vi "Swerve Global Variables.vi"() -> ()   [LabVIEW 2020]
doc: "Global variables in charge of the Swerve Drive subsystem."
panel:
  in  "Target Extension":dbl
  in  "Clamp":dbl
  in  "Manual Rotate In/Out":dbl
  in  "Manual Extend/Retract":dbl
  in  "Reset Gyro":bool
  in  "Use Field Oriented Controls":bool
  in  "Gyro Angle":dbl
  in  "Twist Axis":dbl
  in  "Y Axis":dbl
  in  "X Axis":dbl
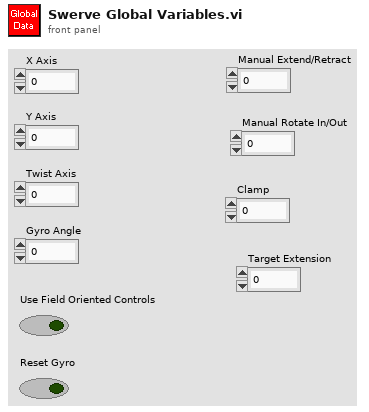
[diagram p1: front panel]
diagram:
